vi "Get Channel (Green).vi"(8 "error in (no error)":errorcluster, 10 "Greyscale Image Destination":T1, 11 "ARGB Image Source":T2) -> (0 "error out":errorcluster, 3 "Greyscale Image Destination (Duplicate)":T1)   [LabVIEW 2020, in "g_ar_toolkit.image.lvlib"]
uses:
  g_ar_toolkit.image.lvlib
  Greyscale Image.ctl
  ARGB Image.ctl
  ExtractOptions.ctl
  g_ar_toolkit.common/Module Path.vi
  <vilib>/Utility/error.llb/Error Cluster From Error Code.vi
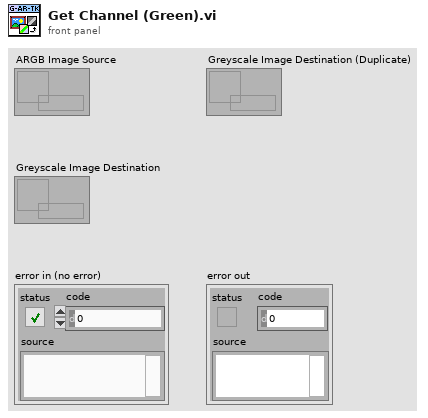
[diagram p1: front panel]
types:
  T1 = typedef "g_ar_toolkit.image.lvlib/Greyscale Image.ctl" = refnum<data-value>
  T2 = typedef "g_ar_toolkit.image.lvlib/ARGB Image.ctl" = refnum<data-value>
  T3 = typedef "g_ar_toolkit.image.lvlib/ExtractOptions.ctl" = enum8{"Blue", "Green", "Red", "Alpha", "Greyscale"}
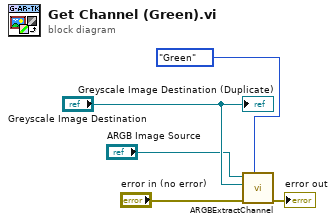
[diagram p0: block diagram]
diagram:
  n1 = call "ARGBExtractChannel.vi"("ExtractOperation"=ExtractOptions."Green" ("Extract_Operation"), "error in (no error)"="error in (no error)", "Greyscale Image Destination"="Greyscale Image Destination", "ARGB Image Source"="ARGB Image Source") -> ("error out"=→"error out":errorcluster)  [unwired: 7 in]
  "Greyscale Image Destination (Duplicate)" <- "Greyscale Image Destination"
